vi "PSA-MaskArray.vi"() -> ()   [LabVIEW 2018]
uses:
  <vilib>/Utility/file.llb/Write Delimited Spreadsheet (DBL).vi
panel:
  in  "tofile(t)":bool
  out "Array 3":dbl[][](array[numeric])
  in  "Freq(GHZ)":dbl[](array[numeric])
  in  "Array 2":dbl[](array[numeric])
  out "Array":dbl[][](array[numeric])
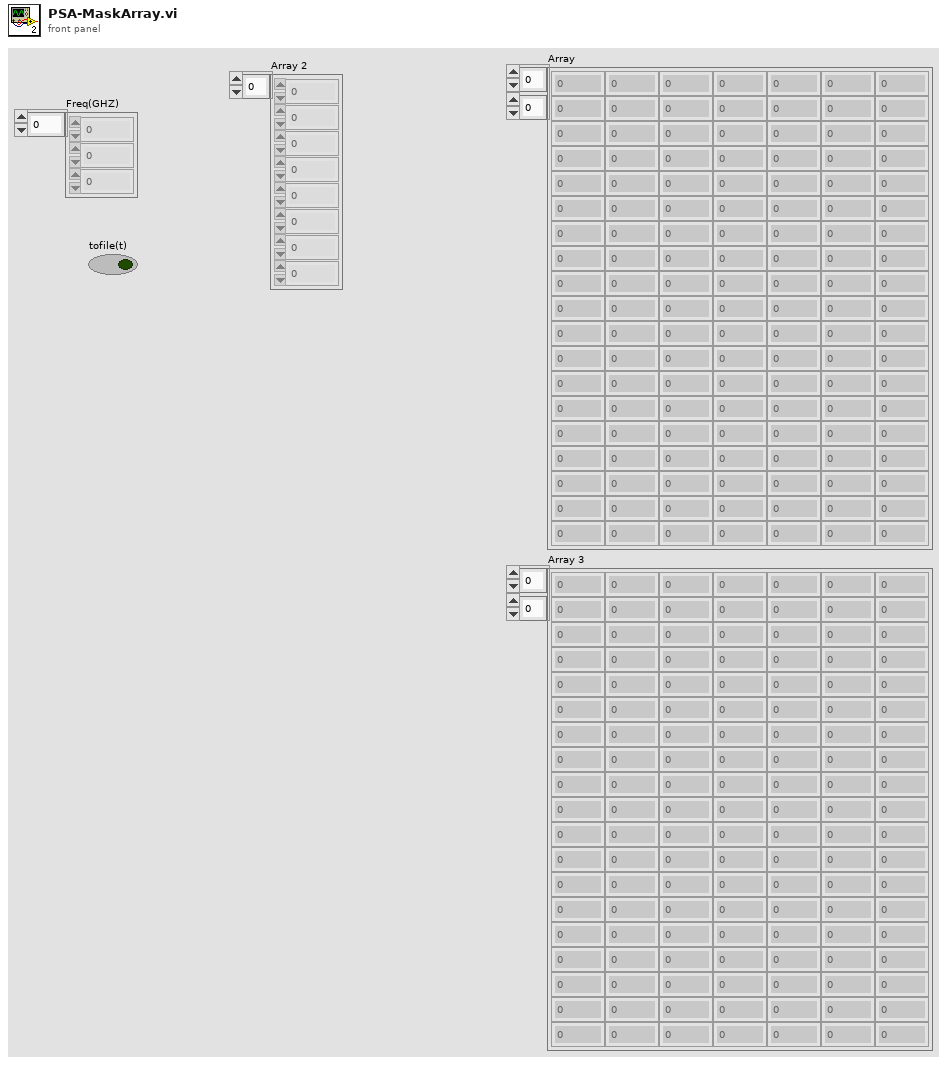
[diagram p1: front panel]
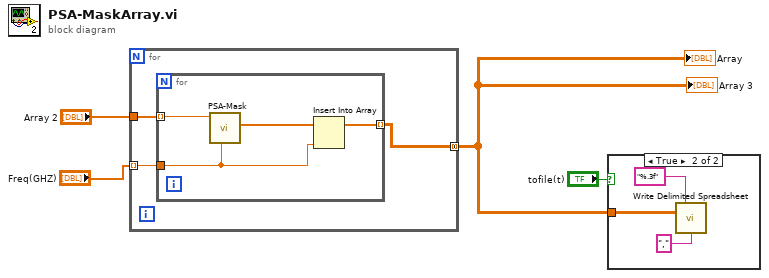
[diagram p0: block diagram]
diagram:
  n1 = for {
    tunnel: "Array 2" -> [w6]
    tunnel: "Freq(GHZ)" -> [w5] mode=indexing
    tunnel: [w7] -> w2 mode=concatenating
    n2 = for {
      tunnel: [w9] -> w7 mode=indexing
      tunnel: w6 -> [w10] mode=indexing
      tunnel: w5 -> [w8]
      n3 = call "PSA-Mask.vi"("Freq(GHZ)"=w8, "Att"=w10) -> ("Array"=w11:dbl[])  [unwired: 7 in, 2 out]
      n4 = Insert Into Array(array=w11, new element=w8) -> (w9:dbl[])  [unwired: 1 in]
    }
  }
  "Array" <- w2
  "Array 3" <- w2
  n5 = case shown="True" "tofile(t)" {
    tunnel: w2 -> [_ w12]
    frame False {
    }
    frame True {
      n6 = call-poly <vilib>:"Write Delimited Spreadsheet.vi"("format (%.3f)"="%.3f", "2D data"=w12, "delimiter (\\t)"="," ("delimiter (\\t)")) -> ()  [unwired: 11 in, 2 out]
    }
  }
